vi "BotSpeak.TestCom.vi"(0 "Bot Settings":T1={"Address"="", "Reply EOF"="", "Hardware"="", "Retries"=0, "Timeout"=10, "Open?"=FALSE}, 1 "Termination":string="\r\n") -> (2 "Bot Settings out":T1, 3 "firmware":string="169.254.32.85", 4 "firmware":dbl)   [LabVIEW 2014]
uses:
  <userlib>/botspeak/VIs/Direct/BotSpeak_Control.ctl
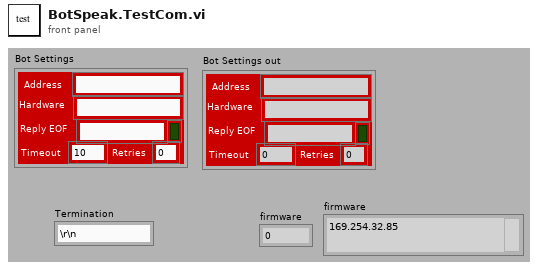
[diagram p1: front panel]
types:
  T1 = typedef "BotSpeak_Control.ctl" = cluster{"Address":string, "Reply EOF":string, "Hardware":string, "Retries":i8, "Timeout":i32, "Open?":bool}
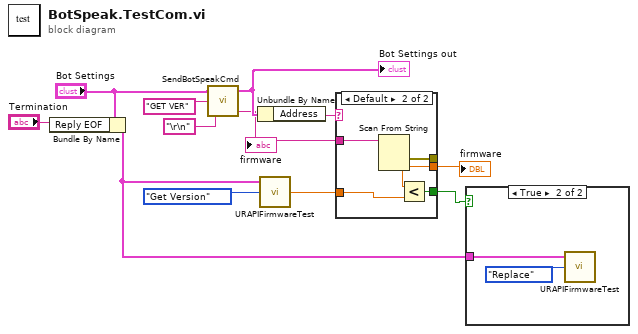
[diagram p0: block diagram]
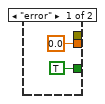
[diagram p3: hidden frame]
diagram:
  n1 = Bundle By Name(cluster="Bot Settings", "Reply EOF"="Termination") -> (w7:T1)
  n2 = call <userlib>:"SendBotSpeakCmd.vi"("Termination"="\r\n", "command"="GET VER", "Last Bot"="Bot Settings") -> ("response"=w1:string, "Bot Settings out"=w4:T1)  [unwired: 1 in]
  "Bot Settings out" <- w4
  "firmware" <- w1
  n3 = Unbundle By Name(w4) -> ("Address"=w6:string)
  n4 = call <userlib>:"URAPIFirmwareTest.vi"("Task"=enum16{"Get Version", "Replace"}."Get Version", "Bot Settings"=w7) -> ("Version"=w8:dbl)  [unwired: 1 in, 2 out]
  n5 = case shown="Default" w6 {
    tunnel: [0.0 w17] -> w11
    tunnel: w1 -> [_ w19]
    tunnel: [_ w18] -> _
    tunnel: [TRUE w16] -> w10
    tunnel: w8 -> [_ w15]
    frame "error" {
    }
    frame Default {
      n6 = Scan From String(input string=w19) -> (error out=w18:errorcluster, output 1=w17:dbl)  [unwired: 4 in, 2 out]
      n7 = Less?(x=w17, y=w15) -> (x < y?=w16:bool)
    }
  }
  "firmware" <- w11
  n8 = case shown="True" w10 {
    tunnel: w7 -> [_ w20]
    frame False {
    }
    frame True {
      n9 = call <userlib>:"URAPIFirmwareTest.vi"("Task"=enum16{"Get Version", "Replace"}."Replace", "Bot Settings"=w20) -> ()  [unwired: 1 in, 3 out]
    }
  }
